vi "_Get or Add Cell.vi"(8 "error in":errorcluster, 10 "Cell Address":string, 11 "Worksheetpart in":refnum<k24>) -> (0 "error out":errorcluster, 2 "Cell":refnum<k24>, 3 "WorksheetPart out":refnum<k24>)   [LabVIEW 2021, in "Open Xml.lvlib"]
uses:
  Open Xml.lvlib
  D:/git/Open-Xml-LabVIEW/dll/DocumentFormat.OpenXml.dll
  dll/DocumentFormat.OpenXml.dll
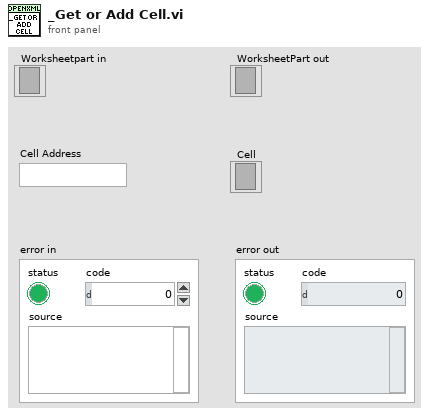
[diagram p1: front panel]
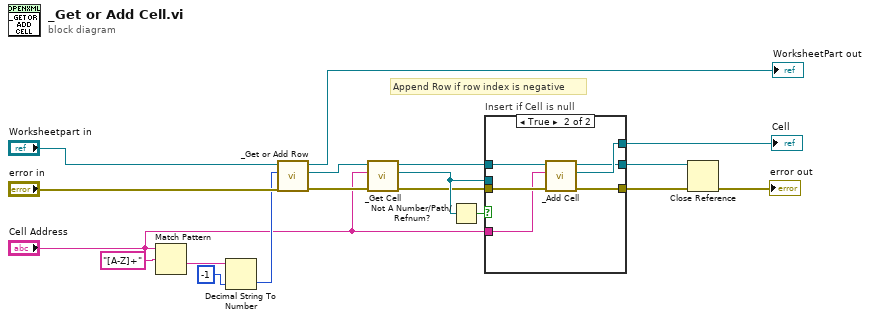
[diagram p0: block diagram]
diagram:
  # "Append Row if row index is negative"
  n1 = Match Pattern(string="Cell Address", regular expression="[A-Z]+") -> (after substring=w13:string)  [unwired: 1 in, 3 out]
  n2 = Decimal String To Number(string=w13, default (0L)=i64 -1 ("default (0 I32)")) -> (number=w11:i64)  [unwired: 1 in, 1 out]
  n3 = call "_Get or Add Row.vi"("error in"="error in", "Row Index"=w11, "Worksheetpart in"="Worksheetpart in") -> ("error out"=w9:errorcluster, "Row"=w10:refnum<k24>, "WorksheetPart out"=→"WorksheetPart out":refnum<k24>)  [unwired: 6 in]
  n4 = call "_Get Cell.vi"("error in"=w9, "Cell Address"="Cell Address", "Row in"=w10) -> ("error out"=w6:errorcluster, "Cell"=w8:refnum<k24>, "Row out"=w5:refnum<k24>)  [unwired: 6 in]
  n5 = Not A Number/Path/Refnum?(number/path/refnum=w8) -> (NaN/Path/Refnum?=w18:bool)
  n6 = case "Insert if Cell is null" shown="True" w18 {
    tunnel: w6 -> [w21 w27]
    tunnel: [w21 w26] -> w3
    tunnel: [w20 w23] -> w17
    tunnel: w8 -> [w20 _]
    tunnel: w5 -> [w19 w25]
    tunnel: "Cell Address" -> [_ w24]
    tunnel: [w19 w22] -> w1
    frame False {
    }
    frame True {
      n7 = call "_Add Cell.vi"("error in"=w27, "Cell Address"=w24, "Row in"=w25) -> ("error out"=w26:errorcluster, "Cell"=w23:refnum<k24>, "Row out"=w22:refnum<k24>)  [unwired: 6 in]
    }
  }
  "Cell" <- w17
  n8 = Close Reference(reference=w1, error in (no error)=w3) -> (error out=→"error out":errorcluster)
